vi "Inject_new Calibration file name.vi"() -> (0 "error out":errorcluster, 4 "Examining:":path)   [LabVIEW 2017]
panel:
  out "Files":dbl
  out "Edits":dbl
  in  "FolderContainingCalibrations":path
  in  "RawDataFoldersToAdjust":path[](array[path])
  in  "Calibration file label":string="An ch 1 Calib filename" caption="Calibration file label (copy from Raw Data File needing correction)"
  in  "Calibration File to be replaced":string="E:\\Enflo_Data_Local\\2018\\EnFlo_Tunnel\\Zoe_Ansell\\Calibrations\\Cal_04-2018\\FFID_Calib_28_03_2018.xls" caption="Calibration File to be replaced  (copy from Raw Data File needing correction)"
  out "CalFilesFound":string[](array[string])
  out "CalFileTimes":dbl[](array[numeric]) format="%#.0f"
  out "File Changed":bool
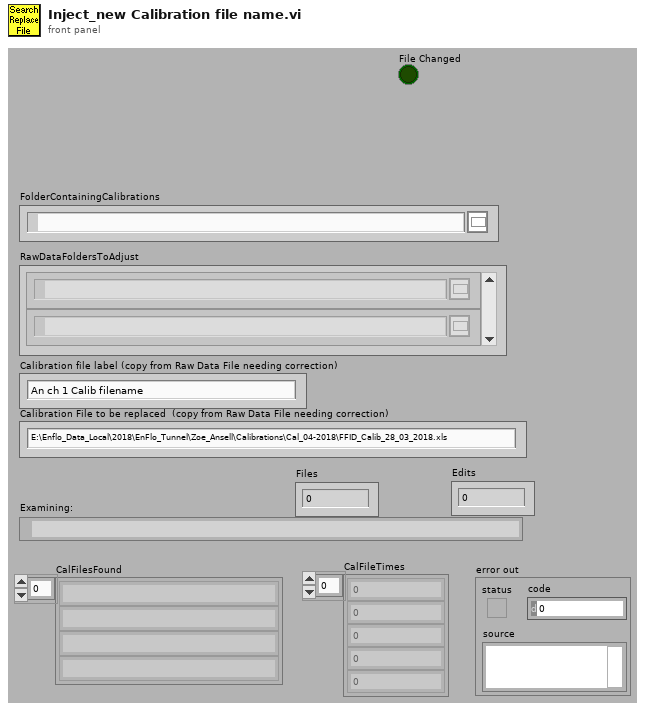
[diagram p1: front panel]
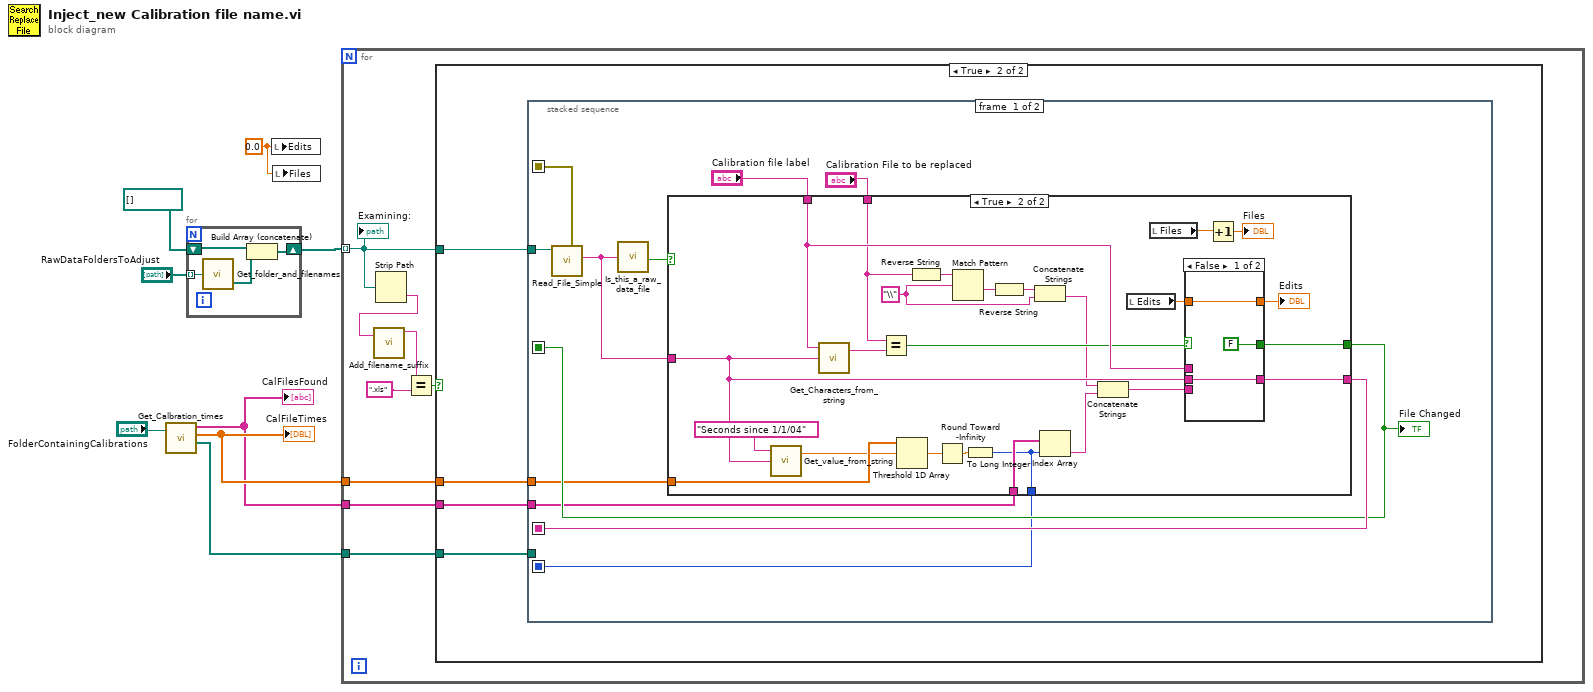
[diagram p0: block diagram]
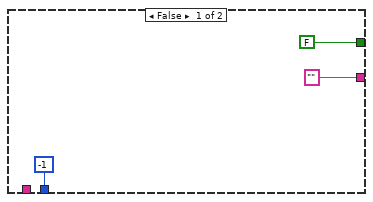
[diagram p3: hidden frame]
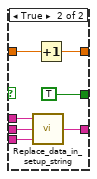
[diagram p4: hidden frame]
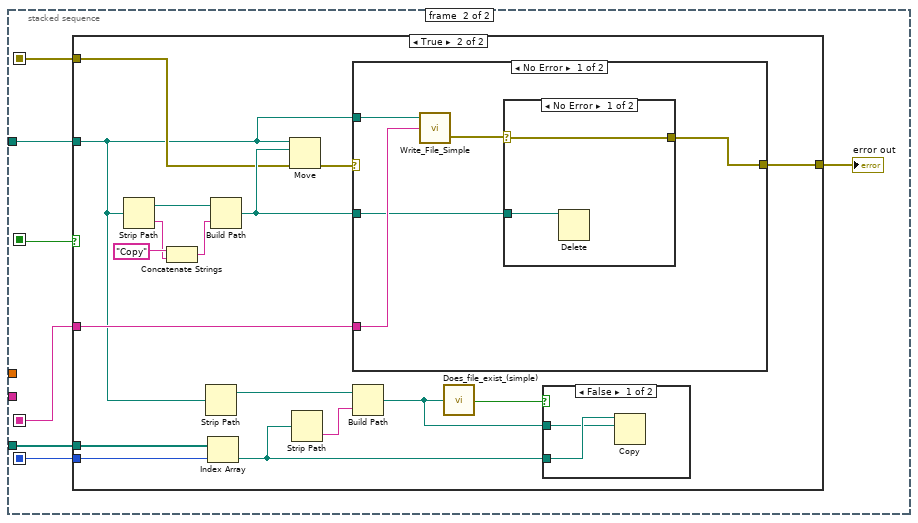
[diagram p5: hidden frame]
diagram:
  w4 = 0.0 ("Edits")
  n1 = call "Get_Calbration_times.vi"("File Path Control"="FolderContainingCalibrations") -> ("CalNames"=w6:string[], "CalTimes"=w8:dbl[], "CalPaths"=w5:path[])  [unwired: 1 in, 1 out]
  "CalFileTimes" <- w8
  "CalFilesFound" <- w6
  n2 = for {
    tunnel: "RawDataFoldersToAdjust" -> [w12] mode=indexing
    shift-right: [w9] -> w2
    shift-left: path[] [] -> [w11]
    n3 = call "Get_folder_and_filenames.vi"("file path (dialog if empty)"=w12) -> ("Files"=w10:path[])  [unwired: 1 out]
    n4 = Build Array (concatenate)(w11, w10) -> (w9:path[])
  }
  n5 = local write "Edits"(w4) -> ()
  n6 = local write "Files"(w4) -> ()
  n7 = for {
    tunnel: w2 -> [w20] mode=indexing
    tunnel: w8 -> [w15]
    tunnel: w6 -> [w14]
    tunnel: w5 -> [w13]
    n8 = Strip Path(path=w20) -> (name=w19:string)  [unwired: 1 out]
    n9 = call "Add_filename_suffix.vi"("Filename"=w19) -> ("Original Suffix"=w18:string)  [unwired: 1 in, 3 out]
    n10 = Equal?(x=w18, y=".xls" ("x")) -> (x = y?=w17:bool)
    n11 = case shown="True" w17 {
      tunnel: w20 -> [_ w24]
      tunnel: w15 -> [_ w23]
      tunnel: w14 -> [_ w22]
      tunnel: w13 -> [_ w21]
      frame False {
      }
      frame True {
        n12 = stacked-sequence {
          seq-local: [w34 _] -> [_ w77]
          seq-local: [w33 _] -> [_ w78]
          seq-local: [w32 _] -> [_ w76]
          seq-local: [w27 _] -> [_ w74]
          tunnel: w24 -> [w35 w80]
          tunnel: w23 -> [w29 _]
          tunnel: w22 -> [w28 _]
          tunnel: w21 -> [_ w75]
          frame #0 {
            n13 = call "Read_File_Simple.vi"("Filename"=w35) -> ("error out"=w34:errorcluster, "string"=w31:string)  [unwired: 4 in, 4 out]
            n14 = call "Is_this_a_raw_data_file.vi"("character string"=w31) -> ("Raw Dat File?"=w30:bool)  [unwired: 2 out]
            n15 = case shown="True" w30 {
              tunnel: "Calibration file label" -> [_ w62]
              tunnel: ["" ("string") w63] -> w33
              tunnel: [FALSE w61] -> w32
              tunnel: w31 -> [_ w60]
              tunnel: "Calibration File to be replaced" -> [_ w44]
              tunnel: w29 -> [_ w56]
              tunnel: w28 -> [_ w53]
              tunnel: [-1 w50] -> w27
              frame False {
              }
              frame True {
                w45 = "\\" ("regular expression")
                n16 = call "Get_value_from_string.vi"("Input string"=w60, "Variable name"="Seconds since 1/1/04") -> ("Value"=w55:dbl)  [unwired: 1 in, 1 out]
                n17 = call "Get_Characters_from_string.vi"("Input string"=w60, "Variable name"=w62) -> ("Value"=w58:string)  [unwired: 1 in, 1 out]
                n18 = Equal?(x=w44, y=w58) -> (x = y?=w57:bool)
                n19 = Threshold 1D Array(2:w55, 3:w56) -> (0:w54:dbl)  [unwired: 1 in]
                n20 = Reverse String(1:w44) -> (0:w48:string)
                n21 = Round Toward -Infinity(1:w54) -> (0:w51:dbl)
                n22 = Match Pattern(string=w48, regular expression=w45) -> (after substring=w47:string)  [unwired: 1 in, 3 out]
                n23 = To Long Integer(number=w51) -> (32bit integer=w50:i32)
                n24 = Reverse String(1:w47) -> (0:w46:string)
                n25 = Concatenate Strings(w46, w45) -> (w43:string)
                n26 = Index Array(array=w53, index=w50) -> (element=w52:string)
                n27 = Concatenate Strings(w43, w52) -> (w49:string)
                n28 = local read "Edits"() -> (w40:dbl)
                n29 = local read "Files"() -> (w41:dbl)
                n30 = case shown="False" w57 {
                  tunnel: w62 -> [_ w73]
                  tunnel: w60 -> [w66 w72]
                  tunnel: [w66 w69] -> w63
                  tunnel: w49 -> [_ w71]
                  tunnel: [FALSE TRUE] -> w61
                  tunnel: w40 -> [w64 w68]
                  tunnel: [w64 w67] -> w39
                  frame False {
                  }
                  frame True {
                    n31 = call "Replace_data_in_setup_string.vi"("New data string"=w71, "Input string"=w72, "Variable name"=w73) -> ("Appended string"=w69:string)
                    n32 = Increment(x=w68) -> (x+1=w67:dbl)
                  }
                }
                "Edits" <- w39
                n33 = Increment(x=w41) -> (x+1=→"Files":dbl)
              }
            }
            "File Changed" <- w32
          }
          frame #1 {
            n34 = case shown="True" w76 {
              tunnel: w80 -> [_ w87]
              tunnel: w78 -> [_ w94]
              tunnel: [w81 w92] -> w79
              tunnel: w77 -> [w81 w90]
              tunnel: w75 -> [_ w89]
              tunnel: w74 -> [_ w88]
              frame False {
              }
              frame True {
                n35 = Strip Path(path=w87) -> (stripped path=w95:path, name=w97:string)
                n36 = Concatenate Strings("Copy" ("name or relative path"), w97) -> (w96:string)
                n37 = Strip Path(path=w87) -> (stripped path=w86:path)  [unwired: 1 out]
                n38 = Index Array(array=w89, index=w88) -> (element=w84:path)
                n39 = Build Path(base path=w95, name or relative path=w96) -> (appended path=w93:path)
                n40 = Move(source path=w87, error in=w90, 10:w93) -> (error out=w91:errorcluster)  [unwired: 2 in, 2 out]
                n41 = Strip Path(path=w84) -> (name=w85:string)  [unwired: 1 out]
                n42 = case shown="No Error" w91 {
                  selector: w91 -> [_ w109]
                  tunnel: w87 -> [w105 _]
                  tunnel: w94 -> [w104 _]
                  tunnel: w93 -> [w103 _]
                  tunnel: [w101 w109] -> w92
                  frame No Error {
                    n43 = call "Write_File_Simple.vi"("character string"=w104, "file path"=w105) -> ("error out"=w102:errorcluster)  [unwired: 1 in, 1 out]
                    n44 = case shown="No Error" w102 {
                      selector: w102 -> [w106 w108]
                      tunnel: w103 -> [w107 _]
                      tunnel: [w106 w108] -> w101
                      frame No Error {
                        n45 = Delete(path (use dialog)=w107) -> ()  [unwired: 4 in, 3 out]
                      }
                      frame Error {
                      }
                    }
                  }
                  frame Error {
                  }
                }
                n46 = Build Path(base path=w86, name or relative path=w85) -> (appended path=w83:path)
                n47 = call "Does_file_exist_(simple).vi"("Pathname"=w83) -> ("exists?"=w82:bool)
                n48 = case shown="False" w82 {
                  tunnel: w84 -> [w100 _]
                  tunnel: w83 -> [w99 _]
                  frame False {
                    n49 = Copy(10:w99, 11:w100) -> ()  [unwired: 3 in, 3 out]
                  }
                  frame True {
                  }
                }
              }
            }
            "error out" <- w79
          }
        }
      }
    }
    "Examining:" <- w20
  }
